vi "oa_Get Angular Speed.vi"   [LabVIEW 2017, in "SoundVib_TachProcess.lvlib"]
uses:
  <vilib>/addons/Sound and Vibration/Order Analysis/Tach Process/SoundVib_TachProcess.lvlib
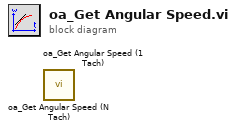
[diagram p0: block diagram]
diagram:
  n1 = call <vilib>:"oa_Get Angular Speed (N Tach).vi"() -> ()  [unwired: 8 in, 4 out]
  n2 = call <vilib>:"oa_Get Angular Speed (1 Tach).vi"() -> ()  [unwired: 8 in, 4 out]
